vi "To Byte.vi"(8 "error in (no error)":errorcluster, 11 "Boolean in":refnum<class "Abs_Boolean.lvclass">) -> (0 "error out":errorcluster, 3 "Boolean out":refnum<class "Abs_Boolean.lvclass">)   [LabVIEW 2021, in "Abs_Boolean.lvclass"]
uses:
  Abs_Boolean.lvclass
panel:
  out "Byte":u8
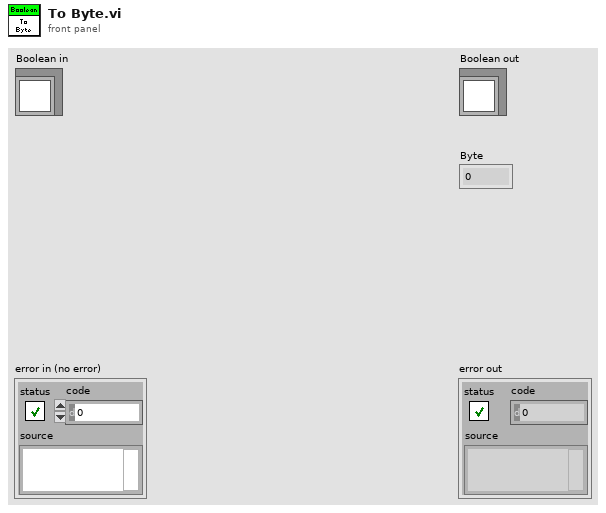
[diagram p1: front panel]
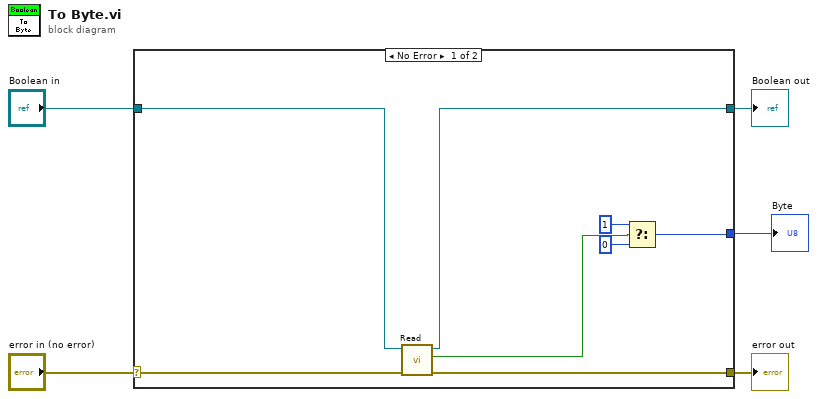
[diagram p0: block diagram]
diagram:
  n1 = case shown="No Error" "error in (no error)" {
    selector: "error in (no error)" -> [w13 w15]
    tunnel: [w12 w15] -> w4
    tunnel: [w10 w14] -> w2
    tunnel: "Boolean in" -> [w11 w14]
    tunnel: [w8 _] -> w1
    frame No Error {
      n2 = call-dynamic "Read.vi"("error in (no error)"=w13, "Boolean in"=w11) -> ("error out"=w12:errorcluster, "Boolean"=w9:bool, "Boolean out"=w10:refnum<class "Abs_Boolean.lvclass">)  [unwired: 7 in]
      n3 = Select(t=u8 1, s=w9, f=u8 0) -> (s? t:f=w8:u8)
    }
    frame Error {
    }
  }
  "error out" <- w4
  "Boolean out" <- w2
  "Byte" <- w1
